vi "Channel Basics Lesson 2.vi"() -> ()   [LabVIEW 2023]
doc: "This VI demonstrates the Stream channel's ability to embed a stop signal in the channel, drawing comparison with the relative complexity (and overall diagram noise) of such code using the queue refnums."
uses:
  <extravilib>/ChannelInstances/Stream-i32/Read With Abort.vi
  <extravilib>/ChannelInstances/Stream-i32/Write With Abort.vi
  <extravilib>/ChannelInstances/Stream-i32/EndpointRead.vi
  <extravilib>/ChannelInstances/Stream-i32/Endpoint.vi
  <extravilib>/ChannelInstances/Stream-i32/Instantiate.vi
  <extravilib>/ChannelInstances/Stream-i32/)Channel.vi
  <resource>/ChannelSupport/_ChannelSupport/WaitIfNeeded.vi
  <extravilib>/ChannelInstances/Stream-i32.lvlib
panel:
  in  "Stop Writer B":bool
  out "Writer B":i32(graph)
  out "Reader B":i32(graph)
  out "Reader A":i32(graph)
  in  "Stop Writer A":bool
  out "Writer A":i32(graph)
  # "Overview: This VI demonstrates how to use channel wires for stopping two parallel loops.\n\nInstructions:\n1. Open the block diagram. Review the lessons presented there.\n2. Run the VI to see that the behavior of the queue implementation (above) is the same as the channel implementation (below). Notice that unlike Lesson 1, in each pair, a single stop button can stop both loops."
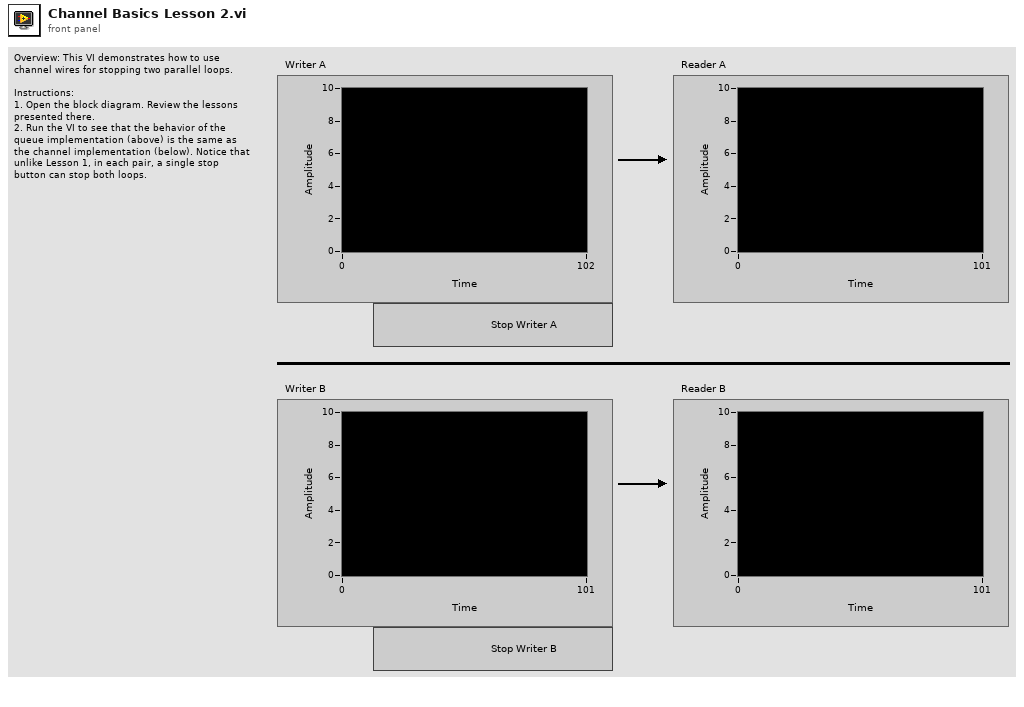
[diagram p1: front panel]
types:
  T1 = typedef "Stream-i32.lvlib/)Channel.ctl" = refnum<queue>
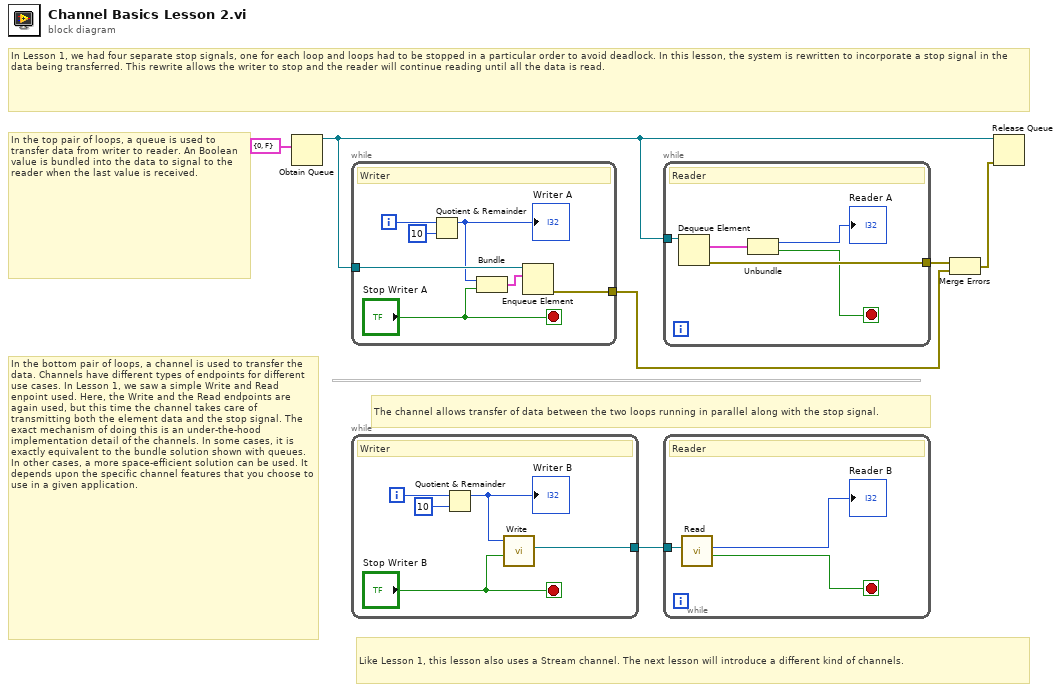
[diagram p0: block diagram]
diagram:
  # "Like Lesson 1, this lesson also uses a Stream channel. The next lesson will introduce a different kind of channels."
  # "In the bottom pair of loops, a channel is used to transfer the data. Channels have different types of endpoints for different use cases. In Lesson 1, we saw a simple Write and Read enpoint used. Here, the Write and the Read endpoints are again used, but this time the channel takes care of transmitting both the element data and the stop signal. The exact mechanism of doing this is an under-the-hood implementation detail of the channels. In some cases, it is exactly equivalent to the bundle solution shown with queues. In other cases, a more space-efficient solution can be used. It depends upon the specific channel features that you choose to use in a given application."
  # "In the top pair of loops, a queue is used to transfer data from writer to reader. An Boolean value is bundled into the data to signal to the reader when the last value is received."
  # "The channel allows transfer of data between the two loops running in parallel along with the stop signal."
  # "In Lesson 1, we had four separate stop signals, one for each loop and loops had to be stopped in a particular order to avoid deadlock. In this lesson, the system is rewritten to incorporate a stop signal in the data being transferred. This rewrite allows the writer to stop and the reader will continue reading until all the data is read."
  n1 = Obtain Queue(element data type=cluster{"element":i32, "last?":bool} {"element"=0, "last?"=FALSE}) -> (queue out=w6:refnum<queue>)  [unwired: 4 in, 2 out]
  n2 = while {
    tunnel: w6 -> [w11]
    tunnel: [w10] -> w4
    i -> [w12]
    stop <- "Stop Writer A" stop-if-true
    # "Writer"
    n3 = Quotient & Remainder(x=w12, y=10) -> (x-y*floor(x/y)=w8:i32)  [unwired: 1 out]
    "Writer A" <- w8
    n4 = Bundle(w8, "Stop Writer A"="Stop Writer A") -> (w7:cluster{i32, "Stop Writer A":bool})  [unwired: 1 in]
    n5 = Enqueue Element(queue=w11, element=w7) -> (error out=w10:errorcluster)  [unwired: 2 in, 2 out]
  }
  n6 = while {
    tunnel: [w15] -> w2
    i -> [w17]
    stop <- "Stop Writer B" stop-if-true
    # "Writer"
    n7 = Quotient & Remainder(x=w17, y=10) -> (x-y*floor(x/y)=w16:i32)  [unwired: 1 out]
    "Writer B" <- w16
    n8 = call <extravilib>:"Write.vi"("last element? (F)"="Stop Writer B", "element"=w16) -> ("channel"=w15:T1)  [unwired: 7 in, 2 out]
  }
  n9 = while {
    tunnel: w6 -> [w23]
    tunnel: [w22] -> w5
    stop <- w19 stop-if-true
    # "Reader"
    n10 = Dequeue Element(queue=w23) -> (element=w21:cluster{"element":i32, "last?":bool}, error out=w22:errorcluster)  [unwired: 2 in, 2 out]
    n11 = Unbundle(w21) -> ("element"=→"Reader A":i32, "last?"=w19:bool)
  }
  n12 = while {
    tunnel: w2 -> [w26]
    stop <- w24 stop-if-true
    # "Reader"
    n13 = call <extravilib>:"Read.vi"("channel"=w26) -> ("last element?"=w24:bool, "element"=→"Reader B":i32)  [unwired: 6 in, 3 out]
  }
  n14 = Merge Errors(w5, w4) -> (w3:errorcluster)
  n15 = Release Queue(queue=w6, error in (no error)=w3) -> ()  [unwired: 1 in, 3 out]
